vi "niRFUtil ERR Check Valid Input (complex wfm).vi"(8 "error in (no error)":errorcluster, 10 "Waveform Name":string="Waveform", 11 "Complex Waveform (In)":T1 {"y" format="%.2f"; "dx" format="%^.2e"; "x0" format="%^.2e"}) -> (0 "error out":errorcluster, 3 "Complex Waveform (Out)":T1 {"y" format="%.2f"; "dx" format="%^.2e"; "x0" format="%^.2e"})   [LabVIEW 2015, in "niRFUtil.lvlib"]
uses:
  niRFUtil.lvlib
  Includes/niRFUtil INC Complex Waveform.ctl
  Includes/niRFUtil INC Complex Array.ctl
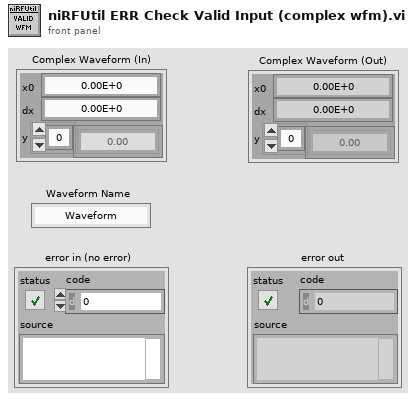
[diagram p1: front panel]
types:
  T1 = typedef "niRFUtil.lvlib/niRFUtil INC Complex Waveform.ctl" = cluster{"x0":dbl, "dx":dbl, "y":T2}
  T2 = typedef "niRFUtil.lvlib/niRFUtil INC Complex Array.ctl" = csg[]
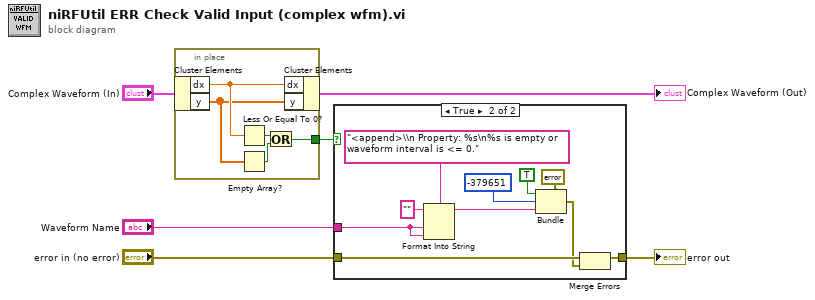
[diagram p0: block diagram]
diagram:
  n1 = in-place {
    in-place-border: [w9] -> w3
    n2 = in-place-cluster #1("Complex Waveform (In)") -> ("dx"=w8:dbl, "y"=w7:T2)
    n3 = Less Or Equal To 0?(x=w8) -> (x <= 0?=w11:bool)
    n4 = Empty Array?(array=w7) -> (empty?=w10:bool)
    n5 = Or(x=w11, y=w10) -> (x .or. y?=w9:bool)
    n6 = in-place-cluster #1("dx"=w8, "y"=w7) -> (→"Complex Waveform (Out)":T1)
  }
  n7 = case shown="True" w3 {
    tunnel: "error in (no error)" -> [w12 w14]
    tunnel: [w12 w15] -> w5
    tunnel: "Waveform Name" -> [_ w20]
    frame False {
    }
    frame True {
      n8 = Format Into String(format string="<append>\\n Property: %s\n%s is empty or waveform interval is <= 0." ("error message (\"\")"), initial string="", w20, w20) -> (resulting string=w18:string)  [unwired: 1 in, 1 out]
      n9 = Bundle(cluster=cluster{"status":bool, i32, string} {"status"=FALSE, 0, ""}, "status"=TRUE, -379651, w18) -> (w13:cluster{"status":bool, i32, string})
      n10 = Merge Errors(w14, w13) -> (w15:errorcluster)
    }
  }
  "error out" <- w5
